vi "ProdaNG.ErrorHandler.vi"(6 "dbHandleIn":i32, 7 "Path":path, 8 "error in":errorcluster, 9 "Additional description":string, 11 "output_parameter":i32) -> (0 "error out":errorcluster)   [LabVIEW 2016]
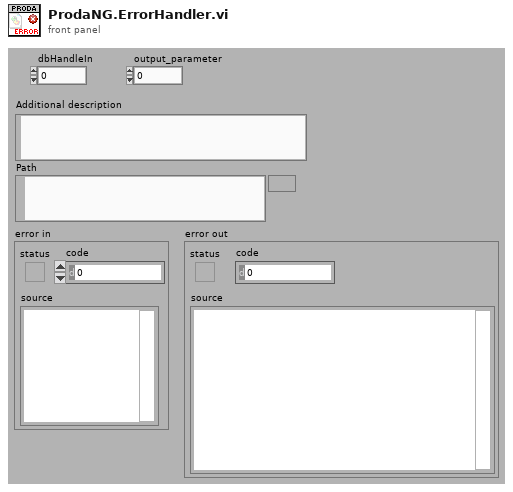
[diagram p1: front panel]
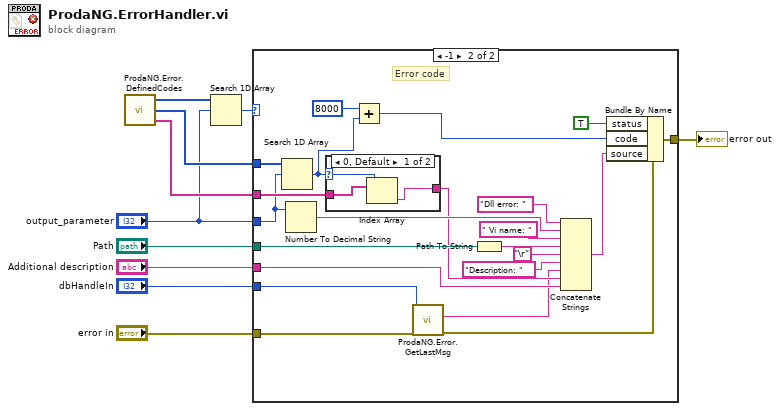
[diagram p0: block diagram]
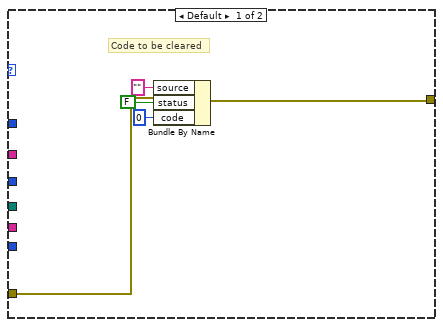
[diagram p2: hidden frame]
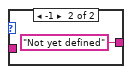
[diagram p3: hidden frame]
diagram:
  n1 = call "ProdaNG.Error.DefinedCodes.vi"() -> ("Defined codes out"=w8:i32[], "Error codes out"=w7:i32[], "Descripotions out"=w6:string[])  [unwired: 5 in]
  n2 = Search 1D Array(1D array=w8, element="output_parameter") -> (index of element=w1:i32)  [unwired: 1 in]
  n3 = case shown="-1" w1 {
    tunnel: "error in" -> [w15 w21]
    tunnel: [w14 w28] -> w9
    tunnel: "output_parameter" -> [_ w23]
    tunnel: "Path" -> [_ w37]
    tunnel: w7 -> [_ w33]
    tunnel: w6 -> [_ w32]
    tunnel: "Additional description" -> [_ w19]
    tunnel: "dbHandleIn" -> [_ w17]
    frame Default {
      # "Code to be cleared"
      n4 = Bundle By Name(cluster=w15, "source"="", "status"=FALSE, "code"=0) -> (w14:errorcluster)
    }
    frame -1 {
      # "Error code"
      n5 = Search 1D Array(1D array=w33, element=w23) -> (index of element=w26:i32)  [unwired: 1 in]
      n6 = Number To Decimal String(number=w23) -> (decimal integer string=w22:string)  [unwired: 1 in]
      n7 = case shown="0, Default" w26 {
        selector: w26 -> [w40 _]
        tunnel: [w38 "Not yet defined" ("string")] -> w18
        tunnel: w32 -> [w39 _]
        frame 0, Default {
          n8 = Index Array(array=w39, index=w40) -> (element=w38:string)
        }
        frame -1 {
        }
      }
      n9 = Add(x=i16 8000, y=w26) -> (x+y=w25:i32)
      n10 = call "ProdaNG.Error.GetLastMsg.vi"("error in"=w21, "dbHandleIn"=w17) -> ("error out"=w20:errorcluster, "Last Error Message"=w16:string)  [unwired: 8 in]
      n11 = Path To String(path=w37) -> (string=w36:string)
      n12 = Concatenate Strings("Dll error: " ("string"), w22, " Vi name: " ("string"), w36, "\r", "Description: " ("string"), w16, w18, w19) -> (w31:string)
      n13 = Bundle By Name(cluster=w20, "status"=TRUE, "code"=w25, "source"=w31) -> (w28:errorcluster)
    }
  }
  "error out" <- w9
